vi "V4.2校准列表读取.vi"(8 "error in (no error)":errorcluster, 9 "量程":enum16{"低量程", "高量程"}(ring), 10 "测量模式":T2(ring), 11 "测量参数":u16(ring) items=["总磷"=1, "总氮"=2, "氨氮"=3, "COD"=22]) -> (0 "error out":errorcluster, 3 "校准参数 out":T1 {"拟合方法" items=["线性", "多项式", "折线"]})   [LabVIEW 2016, in "斯坦道通用流路CODmn.lvlib"]
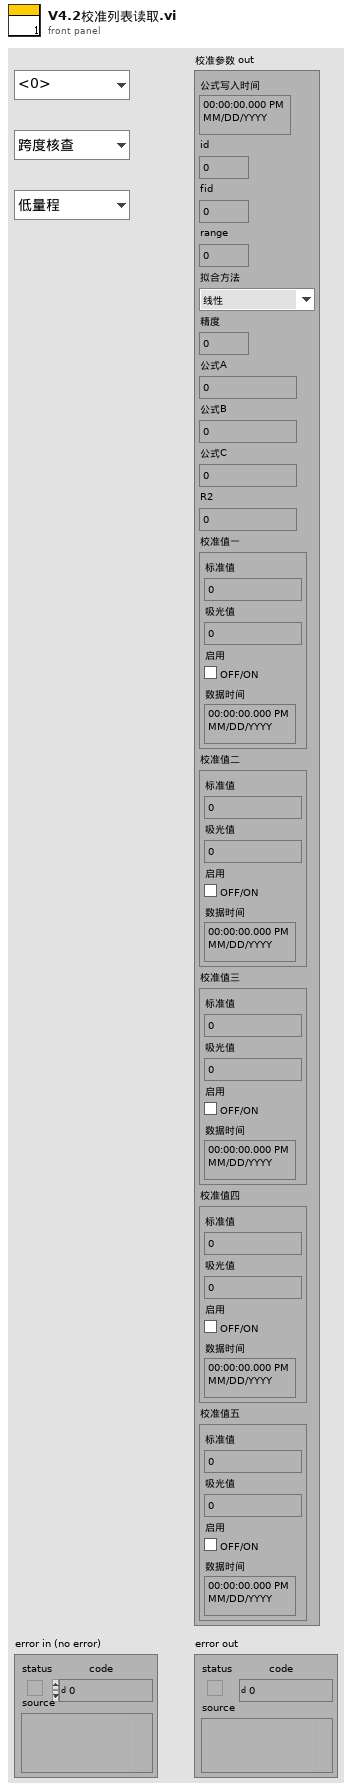
[diagram p1: front panel]
types:
  T1 = typedef "斯坦道通用流路CODmn.lvlib/校准参数.ctl" = cluster{"公式写入时间":timestamp, "id":u8, "fid":u8, "range":u8, "拟合方法":u16, "精度":u16, "公式A":sgl, "公式B":sgl, "公式C":sgl, "R2":sgl, "校准值一":cluster{"标准值":sgl, "吸光值":sgl, "启用":bool, "数据时间":timestamp}, "校准值二":cluster{"标准值":sgl, "吸光值":sgl, "启用":bool, "数据时间":timestamp}, "校准值三":cluster{"标准值":sgl, "吸光值":sgl, "启用":bool, "数据时间":timestamp}, "校准值四":cluster{"标准值":sgl, "吸光值":sgl, "启用":bool, "数据时间":timestamp}, "校准值五":cluster{"标准值":sgl, "吸光值":sgl, "启用":bool, "数据时间":timestamp}}
  T2 = enum16{"跨度核查", "水样测量", "零点核查", "标样核查", "加标回收", "快捷测试", "空白校准", "标样校准"}
  T3 = typedef "SingleStepTestV3.lvlib/SingleStepTestV3.lvclass/仪器版本.ctl" = enum16{"V3.1版", "V4版", "V3版", "V4.2版"}
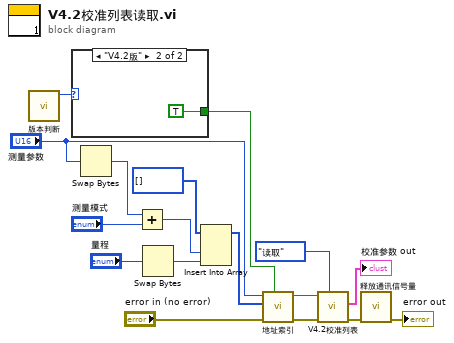
[diagram p0: block diagram]
diagram:
  n1 = call "版本判断.vi"() -> ("仪器版本"=w2:T3)  [unwired: 11 in]
  n2 = case shown="\"V4.2版\"" w2 {
    tunnel: [_ TRUE] -> w1
    frame "V3.1版", Default {
    }
    frame "V4.2版" {
    }
  }
  n3 = Swap Bytes(anything="测量参数") -> (byte swapped=w15:u16)
  n4 = Add(x=w15, y="测量模式") -> (x+y=w17:u16)
  n5 = Swap Bytes(anything="量程") -> (byte swapped=w14:u16)
  n6 = Insert Into Array(array=u16[] [] ("数组"), new element #1=w17, new element #2=w14) -> (w13:u16[])  [unwired: 1 in]
  n7 = call "地址索引.vi"("4.2写公式？"=w1, "error in (no error)"="error in (no error)", "values"=w13, "测量参数"="测量参数") -> ("error out"=w10:errorcluster, "MB session out"=w11:refnum<class "MB_Master.lvclass">)  [unwired: 6 in]
  n8 = call "V4.2校准列表.vi"("功能"=enum16{"读取", "写入"}."读取", "error in (no error)"=w10, "MB session in"=w11) -> ("error out"=w8:errorcluster, "校准参数 out"=→"校准参数 out":T1)  [unwired: 6 in, 1 out]
  n9 = call "释放通讯信号量.vi"("error in (no error)"=w8) -> ("error out"=→"error out":errorcluster)  [unwired: 10 in]
